vi "Database Command Get Parameters.vi"(8 "error in (no error)":errorcluster caption="错误输入（无错误）", 11 "Database Command 输入":refnum<class "Database Command.lvclass"> caption="DNL_LabVIEW Object in") -> (0 "error out":errorcluster caption="错误输出", 1 "parameters":T1[](array[typedef]), 3 "Database Command 输出":refnum<class "Database Command.lvclass"> caption="DNL_LabVIEW Object out")   [LabVIEW 2011, in "Database Command.lvclass"]
uses:
  Database Command.lvclass
  <vilib>/addons/database/Auxilliary.llb/DB Tools Parameter Info.ctl
  <vilib>/addons/database/Auxilliary.llb/DB Tools DataTypes.ctl
  <vilib>/addons/database/Auxilliary.llb/DB Tools Parameter Dir.ctl
  Database Command.lvclass/Database Command.ctl
  <vilib>/addons/database/NI_Database_API.lvlib
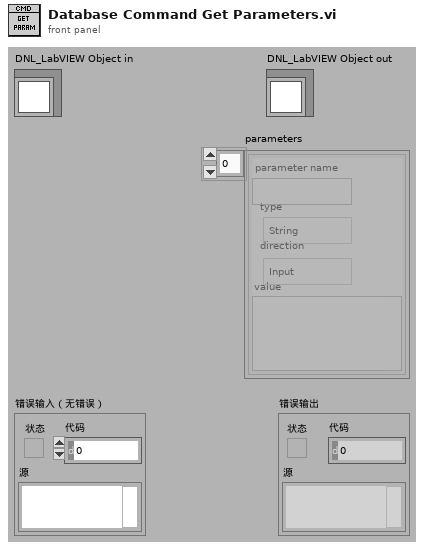
[diagram p1: front panel]
types:
  T1 = typedef "NI_Database_API.lvlib/DB Tools Parameter Info.ctl" = cluster{"parameter name":string, "type":T2, "direction":T3, "value":variant}
  T2 = typedef "NI_Database_API.lvlib/DB Tools DataTypes.ctl" = enum16{"String", "Long (I32)", "Single (SGL)", "Double (DBL)", "Date/Time", "Binary"}
  T3 = typedef "NI_Database_API.lvlib/DB Tools Parameter Dir.ctl" = enum32{"Input", "Output", "Input/Output", "Return Value"}
  T4 = cluster{"Name":string, "data type":T2, "direction":T3, "Value":variant}
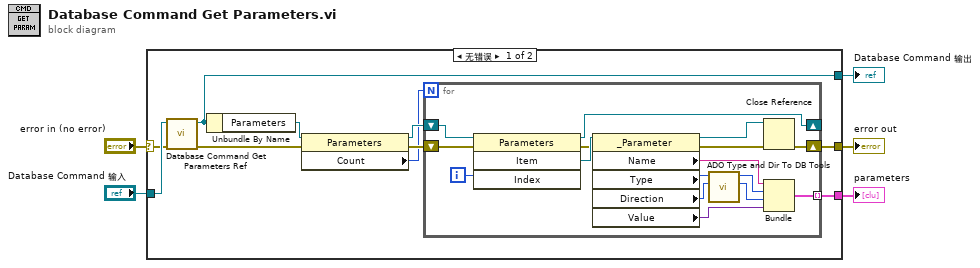
[diagram p0: block diagram]
diagram:
  n1 = case shown="无错误" "error in (no error)" {
    selector: "error in (no error)" -> [w14 w33]
    tunnel: [w7 w33] -> w4
    tunnel: [w13 w32] -> w2
    tunnel: "Database Command 输入" -> [w15 w32]
    tunnel: [w8 _] -> w1
    frame No Error {
      n2 = call "Database Command Get Parameters Ref.vi"("error in (no error)"=w14, "Database Command 输入"=w15) -> ("error out"=w11:errorcluster, "Database Command 输出"=w13:refnum<class "Database Command.lvclass">)  [unwired: 8 in]
      n3 = Unbundle By Name(w13) -> ("Parameters"=w12:refnum<k7>)
      n4 = property class="Parameters"(reference=w12, error in=w11) -> (reference out=w10:refnum<k7>, error out=w9:errorcluster, "Count"=w6:i32)
      n5 = for {
        N: w6 -> [_]
        shift-right: [w29] -> _
        shift-left: w10 -> [w16]
        shift-right: [w18] -> w7
        shift-left: w9 -> [w31]
        tunnel: [w20] -> w8 mode=indexing
        i -> [w30]
        n6 = invoke class="Parameters" method="Item"(reference=w16, error in=w31, "Index"=w30) -> (reference out=w29:refnum<k7>, error out=w27:errorcluster, "Item"=w28:refnum<k7>)  [unwired: 1 in, 1 out]
        n7 = property class="_Parameter"(reference=w28, error in=w27) -> (reference out=w17:refnum<k7>, error out=w19:errorcluster, "Name"=w24:string, "Type"=w26:i32, "Direction"=w25:i32, "Value"=w21:variant)
        n8 = call "ADO Type and Dir To DB Tools.vi"("ADO Direction"=w25, "ADO type"=w26) -> ("direction"=w22:T3, "data type"=w23:T2)  [unwired: 7 in, 1 out]
        n9 = Close Reference(reference=w17, error in (no error)=w19) -> (error out=w18:errorcluster)
        n10 = Bundle("Name"=w24, "data type"=w23, "direction"=w22, "Value"=w21) -> (w20:T4)  [unwired: 1 in]
      }
    }
    frame Error {
    }
  }
  "error out" <- w4
  "Database Command 输出" <- w2
  "parameters" <- w1
